vi "TreeItem.Get.vi"(6 "Custom Device Path":string, 8 "error in (no error)":errorcluster, 9 "Tree":T1[](array[typedef]) {"Properties"."Type" items=["K_STRING", "K_BOOL", "K_I32", "K_U32", "K_DOUBLE", "K_U64", "K_VARIANT", "K_DEPENDENTFILE", "K_DEPENDENTNODE", "K_DATASOURCENODE", "K_U16", "K_DBLARR", "K_U32ARR", "K_I32ARR", "K_STRINGARR", "K_DICTIONARY", "K_DICTIONARYARR"]}, 10 "BaseNode Ref":refnum<k39>, 11 "NodeIDUtil Ref":refnum<k39>) -> (0 "error out":errorcluster, 1 "Tree":T1[](array[typedef]) {"Properties"."Type" items=["K_STRING", "K_BOOL", "K_I32", "K_U32", "K_DOUBLE", "K_U64", "K_VARIANT", "K_DEPENDENTFILE", "K_DEPENDENTNODE", "K_DATASOURCENODE", "K_U16", "K_DBLARR", "K_U32ARR", "K_I32ARR", "K_STRINGARR", "K_DICTIONARY", "K_DICTIONARYARR"]}, 2 "BaseNode Ref out":refnum<k39>, 3 "NodeIDUtil Ref out":refnum<k39>)   [LabVIEW 2027, in "Advanced System Definition.lvlib"]
uses:
  SysDef API/Advanced System Definition.lvlib
  <vilib>/NI VeriStand/Custom Device API/Custom Device Channel Type.ctl
  <vilib>/NI VeriStand/Custom Device API/Custom Device API.lvlib
  <vilib>/NI VeriStand/Custom Device API/Custom Device Channel.ctl
  <vilib>/NI VeriStand/Custom Device API/Custom Device Waveform DataType.ctl
  <vilib>/NI VeriStand/Custom Device API/Custom Device Waveform.ctl
  <vilib>/NI/NI VeriStand Advanced SysDef API/_Types/TreeItem.Info.ctl
  _Types/TreeItem.Property.ctl
  _Types/TreeItem.ctl
  C:/NetCoreDLL/NationalInstruments.VeriStand.SystemStorage.dll
  NetCoreDLL/NationalInstruments.VeriStand.SystemStorage.dll
  C:/NetCoreDLL/NationalInstruments.VeriStand.SystemDefinitionAPI.dll
  NetCoreDLL/NationalInstruments.VeriStand.SystemDefinitionAPI.dll
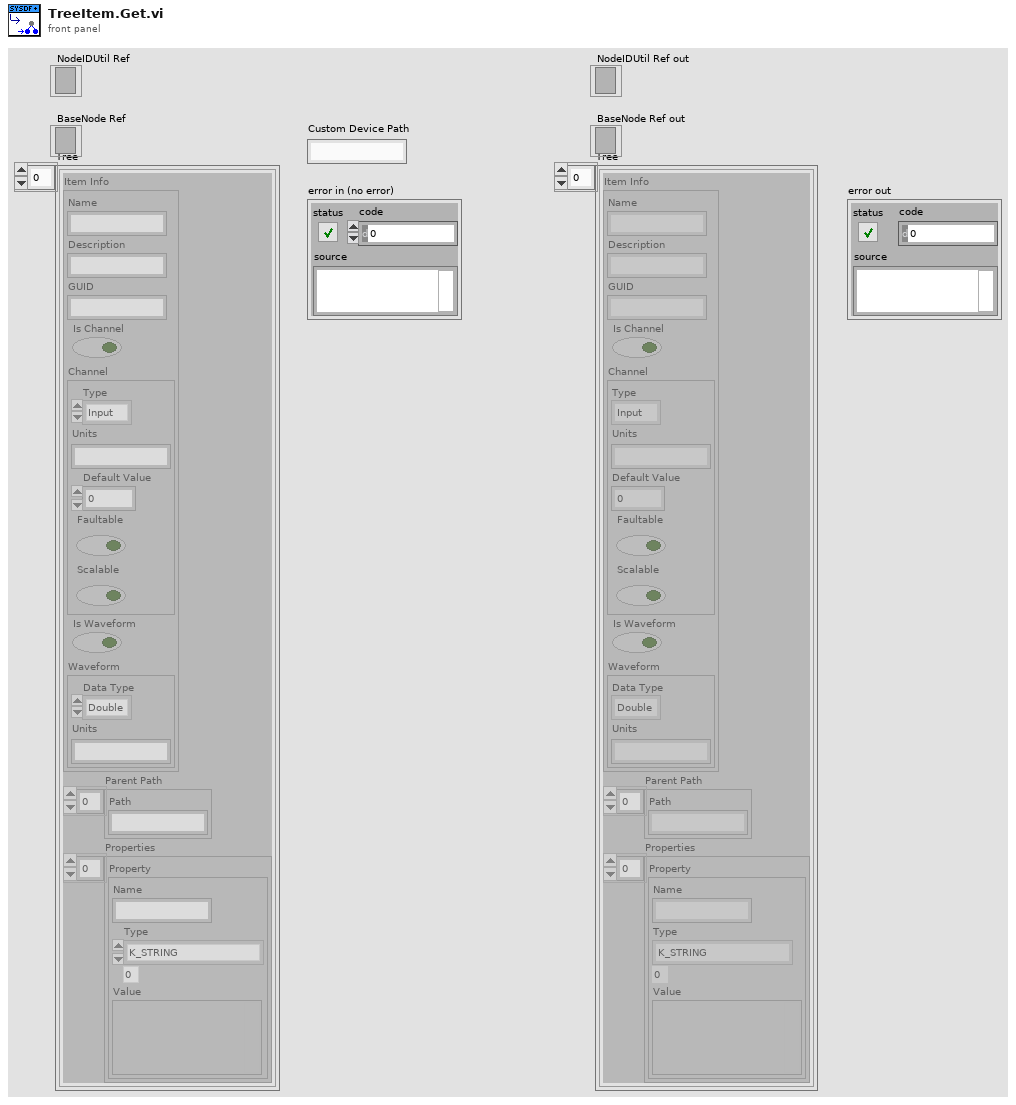
[diagram p1: front panel]
types:
  T1 = typedef "Advanced System Definition.lvlib/TreeItem.ctl" = cluster{"Item Info":T2, "Parent Path":string[], "Properties":T7[]}
  T2 = typedef "Advanced System Definition.lvlib/TreeItem.Info.ctl" = cluster{"Name":string, "Description":string, "GUID":string, "Is Channel":bool, "Channel":T3, "Is Waveform":bool, "Waveform":T5}
  T3 = typedef "Custom Device API.lvlib/Custom Device Channel.ctl" = cluster{"Type":T4, "Units":string, "Default Value":dbl, "Faultable":bool, "Scalable":bool}
  T4 = typedef "Custom Device API.lvlib/Custom Device Channel Type.ctl" = enum16{"Input", "Output"}
  T5 = typedef "Custom Device API.lvlib/Custom Device Waveform.ctl" = cluster{"Data Type":T6, "Units":string}
  T6 = typedef "Custom Device API.lvlib/Custom Device Waveform DataType.ctl" = enum16{"Double", "Complex Double"}
  T7 = typedef "Advanced System Definition.lvlib/TreeItem.Property.ctl" = cluster{"Name":string, "Type":i32, "Value":variant}
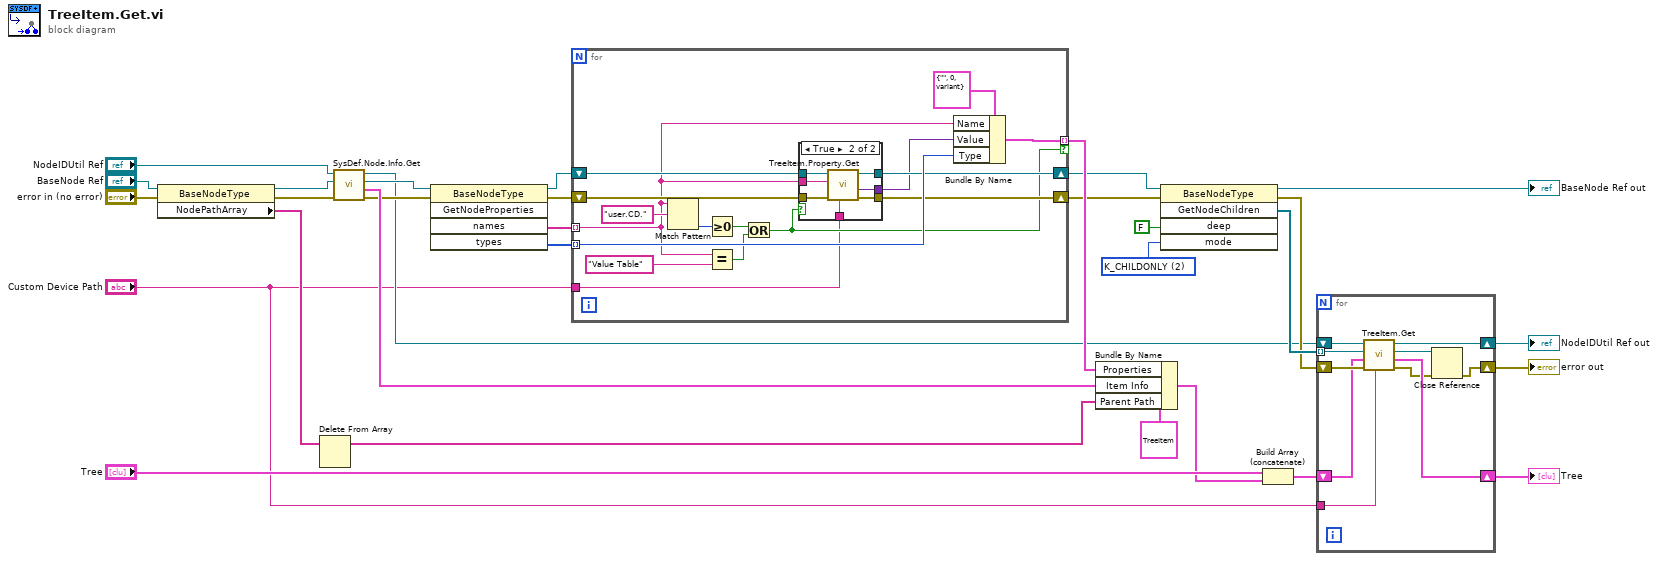
[diagram p0: block diagram]
diagram:
  w18 = 2 items=["K_BFS", "K_DFS", "K_CHILDONLY", "K_UP"] ("mode")
  n1 = property class="BaseNodeType"(reference="BaseNode Ref", error in="error in (no error)") -> (reference out=w6:refnum<k39>, error out=w9:errorcluster, "NodePathArray"=w7:string[])
  n2 = Delete From Array(array=w7) -> (array with subset deleted=w12:string[])  [unwired: 2 in, 1 out]
  n3 = call "SysDef.Node.Info.Get.vi"("error in (no error)"=w9, "NationalInstruments.VeriStand.SystemStorage.BaseNodeType"=w6, "NationalInstruments.VeriStand.SystemDefinitionAPI.NodeIDUtil"="NodeIDUtil Ref") -> ("error out"=w14:errorcluster, "Item Info"=w23:T2, "NationalInstruments.VeriStand.SystemStorage.BaseNodeType"=w5:refnum<k39>, "NationalInstruments.VeriStand.SystemDefinitionAPI.NodeIDUtil"=w4:refnum<k39>)  [unwired: 5 in]
  n4 = invoke class="BaseNodeType" method="GetNodeProperties"(reference=w5, error in=w14) -> (reference out=w25:refnum<k39>, error out=w26:errorcluster, "names"=w28:string[], "types"=w27:i32[])  [unwired: 3 in, 1 out]
  n5 = for {
    tunnel: w27 -> [w42] mode=indexing
    tunnel: w28 -> [w37] mode=indexing
    shift-right: [w38] -> w21
    shift-left: w26 -> [w45]
    tunnel: [w41] -> w22 mode=indexing if=w33
    shift-right: [w40] -> w20
    shift-left: w25 -> [w44]
    tunnel: "Custom Device Path" -> [w32]
    n6 = Match Pattern(string=w37, regular expression="user.CD.") -> (offset past match=w46:i32)  [unwired: 1 in, 3 out]
    n7 = Greater Or Equal To 0?(x=w46) -> (x >= 0?=w34:bool)
    n8 = Equal?(x=w37, y="Value Table") -> (x = y?=w35:bool)
    n9 = Or(x=w34, y=w35) -> (x .or. y?=w33:bool)
    n10 = case shown="True" w33 {
      tunnel: w45 -> [w49 w56]
      tunnel: [w49 w55] -> w38
      tunnel: [_ w54] -> w39
      tunnel: w44 -> [w48 w53]
      tunnel: w37 -> [_ w52]
      tunnel: [w48 w51] -> w40
      tunnel: w32 -> [_ w50]
      frame False {
      }
      frame True {
        n11 = call "TreeItem.Property.Get.vi"("Custom Device Path"=w50, "error in (no error)"=w56, "Property Name"=w52, "NationalInstruments.VeriStand.SystemStorage.BaseNodeType"=w53) -> ("error out"=w55:errorcluster, "Variant"=w54:variant, "NationalInstruments.VeriStand.SystemStorage.BaseNodeType"=w51:refnum<k39>)  [unwired: 4 in, 1 out]
      }
    }
    n12 = Bundle By Name(cluster=T7 {"Name"="", "Type"=0, "Value"=variant(string "")}, "Name"=w37, "Value"=w39, "Type"=w42) -> (w41:T7)
  }
  n13 = Bundle By Name(cluster=T1 {"Item Info"={"Name"="", "Description"="", "GUID"="", "Is Channel"=FALSE, "Channel"={"Type"=enum."Input", "Units"="", "Default Value"=0.0, "Faultable"=FALSE, "Scalable"=FALSE}, "Is Waveform"=FALSE, "Waveform"={"Data Type"=enum."Double", "Units"=""}}, "Parent Path"=[], "Properties"=[]}, "Properties"=w22, "Item Info"=w23, "Parent Path"=w12) -> (w17:T1)
  n14 = invoke class="BaseNodeType" method="GetNodeChildren"(reference=w20, error in=w21, "deep"=FALSE, "mode"=w18) -> (reference out=→"BaseNode Ref out":refnum<k39>, error out=w13:errorcluster, "GetNodeChildren"=w16:refnum<k39>[])  [unwired: 1 in, 2 out]
  n15 = Build Array (concatenate)("Tree", w17) -> (w15:T1[])
  n16 = for {
    tunnel: w16 -> [w63] mode=indexing
    shift-right: [w64] -> w31
    shift-left: w15 -> [w65]
    shift-right: [w59] -> w29
    shift-left: w13 -> [w66]
    shift-right: [w61] -> w11
    shift-left: w4 -> [w62]
    tunnel: "Custom Device Path" -> [w57]
    n17 = call "TreeItem.Get.vi"("Custom Device Path"=w57, "error in (no error)"=w66, "Tree"=w65, "NationalInstruments.VeriStand.SystemStorage.BaseNodeType"=w63, "NationalInstruments.VeriStand.SystemDefinitionAPI.NodeIDUtil"=w62) -> ("error out"=w60:errorcluster, "Tree"=w64:T1[], "NationalInstruments.VeriStand.SystemStorage.BaseNodeType"=w58:refnum<k39>, "NationalInstruments.VeriStand.SystemDefinitionAPI.NodeIDUtil"=w61:refnum<k39>)  [unwired: 3 in]
    n18 = Close Reference(reference=w58, error in (no error)=w60) -> (error out=w59:errorcluster)
  }
  "Tree" <- w31
  "error out" <- w29
  "NodeIDUtil Ref out" <- w11
